vi "Prepare Original and Reply Message.vi"(8 "Error In":errorcluster, 10 "Data Read":string) -> (0 "Error Out":errorcluster, 1 "Reply Message":T1={"Command"="zxcvbnm,", "Data"=["asdfghjk", "qwertyui"], "Script ID"=0, "LabVIEW Server ID"="zxcvbnm,", "Python Message ID"=0}, 2 "Original Message":T1={"Command"="zxcvbnm,", "Data"=["asdfghjk", "qwertyui"], "Script ID"=0, "LabVIEW Server ID"="zxcvbnm,", "Python Message ID"=0}, 3 "Data Payload":string[](array[string]), 5 "\"True\" in Command?":bool, 7 "Command":string)   [LabVIEW 2013, in "TS.lvlib"]
uses:
  TS.lvlib
  LabVIEW Python Connector Message.ctl
panel:
  out "Data":string
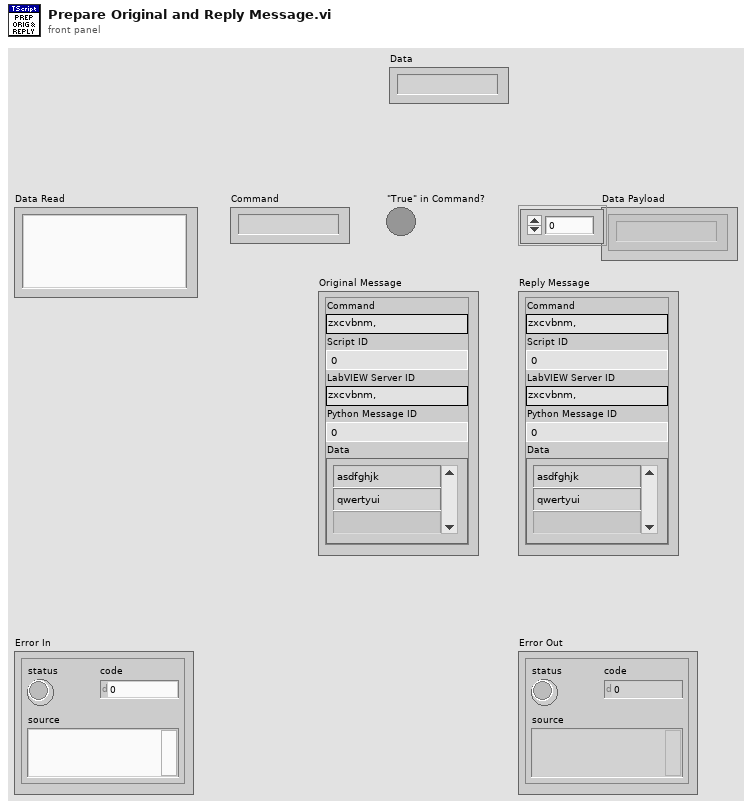
[diagram p1: front panel]
types:
  T1 = typedef "TS.lvlib/LabVIEW Python Connector Message.ctl" = cluster{"Command":string, "Data":string[], "Script ID":i64, "LabVIEW Server ID":string, "Python Message ID":i32}
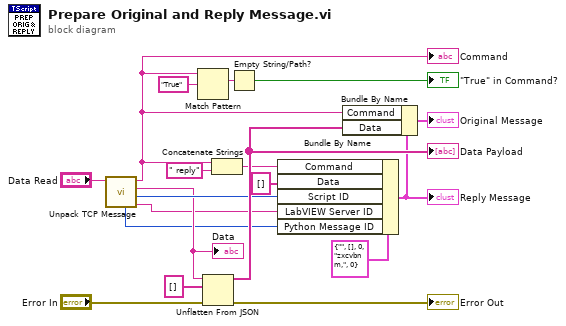
[diagram p0: block diagram]
diagram:
  n1 = call "Unpack TCP Message.vi"("data in"="Data Read") -> ("LabVIEW Server ID"=w2:string, "Script ID"=w15:i64, "Data"=w13:string, "Command"=w16:string, "Python Message ID"=w1:i32)  [unwired: 6 in]
  "Command" <- w16
  "Data" <- w13
  n2 = Match Pattern(string=w16, regular expression="True") -> (match substring=w18:string)  [unwired: 1 in, 3 out]
  n3 = Unflatten From JSON(JSON string=w13, type and defaults=string[] [] ("Data"), error in (no error)="Error In") -> (value=w19:string[], error out=→"Error Out":errorcluster)  [unwired: 4 in]
  "Data Payload" <- w19
  n4 = Concatenate Strings(w16, " reply" ("string")) -> (w10:string)
  n5 = Empty String/Path?(string/path=w18) -> (empty?=→"\"True\" in Command?":bool)
  n6 = Bundle By Name(cluster=T1 {"Command"="", "Data"=[], "Script ID"=0, "LabVIEW Server ID"="zxcvbnm,", "Python Message ID"=0} ("Tcp Message"), "Command"=w10, "Data"=string[] [], "Script ID"=w15, "LabVIEW Server ID"=w2, "Python Message ID"=w1) -> (w6:T1)
  "Reply Message" <- w6
  n7 = Bundle By Name(cluster=w6, "Command"=w16, "Data"=w19) -> (→"Original Message":T1)
